vi "nominal asset search.vi"(0 "client":i32, 1 "property_value":string, 2 "out_count":u32, 5 "search_text":string, 7 "label":string, 9 "property_key":string, 11 "error in (no error)":errorcluster, 12 "out_list":i32) -> (4 "out_count out":u32, 6 "function return":i32, 14 "out_list out":i32, 15 "error out":errorcluster)   [LabVIEW 2020, in "client.lvlib"]
doc: "int32_t nominal_asset_search(int32_t client,\n const char *search_text,\n const char *label,\n const char *property_key,\n const char *property_value,\n int32_t *out_list,\n uint32_t *out_count);"
uses:
  client.lvlib
  nominalClient_64.dll
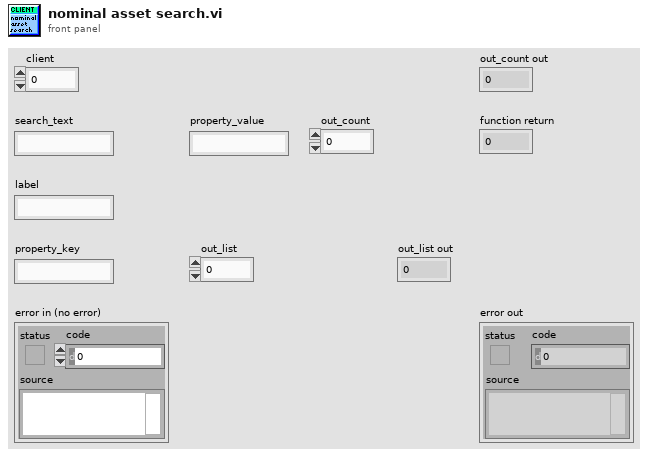
[diagram p1: front panel]
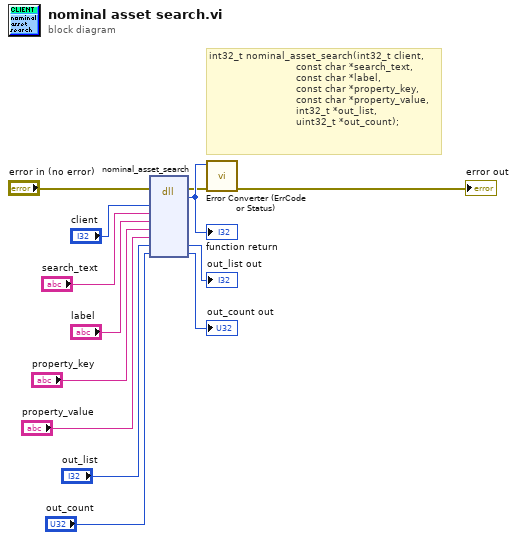
[diagram p0: block diagram]
diagram:
  # "int32_t nominal_asset_search(int32_t client,\n                             const char *search_text,\n                             const char *label,\n                             const char *property_key,\n                             const char *property_value,\n                             int32_t *out_list,\n                             uint32_t *out_count);"
  n1 = dll-call lib="C:/code/labview-client-rs/lv_src/client/nominalClient_*.dll" fn="nominal_asset_search"(error in="error in (no error)", "client"="client", "search_text"="search_text", "label"="label", "property_key"="property_key", "property_value"="property_value", "out_list"="out_list", "out_count"="out_count") -> (error out=w2:errorcluster, w13:i32, "out_list"=→"out_list out":i32, "out_count"=→"out_count out":u32)  [unwired: 7 in, 1 out]
  "function return" <- w13
  n2 = call "Error Converter (ErrCode or Status).vi"("error in (no error)"=w2, "error code"=w13) -> ("error out"=→"error out":errorcluster)  [unwired: 9 in]
